vi "Replace-action.vi"(8 "error in (no error)":errorcluster, 9 "Position in":i32, 10 "Action":refnum<class "Action.lvclass">, 11 "Sequence in":refnum<class "Action-sequence.lvclass">) -> (0 "error out":errorcluster, 1 "Position":i32, 2 "Replaced action":refnum<class "Action.lvclass">, 3 "Sequence out":refnum<class "Action-sequence.lvclass">)   [LabVIEW 2013, in "PowderDeposition.lvlib" / "Action-sequence.lvclass"]
uses:
  Action-sequence.lvclass
  Action/Action.lvclass
  Action-sequence.lvclass/Action-sequence.ctl
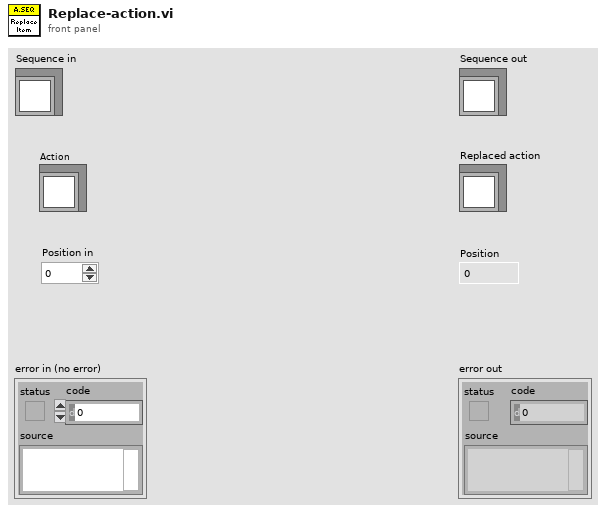
[diagram p1: front panel]
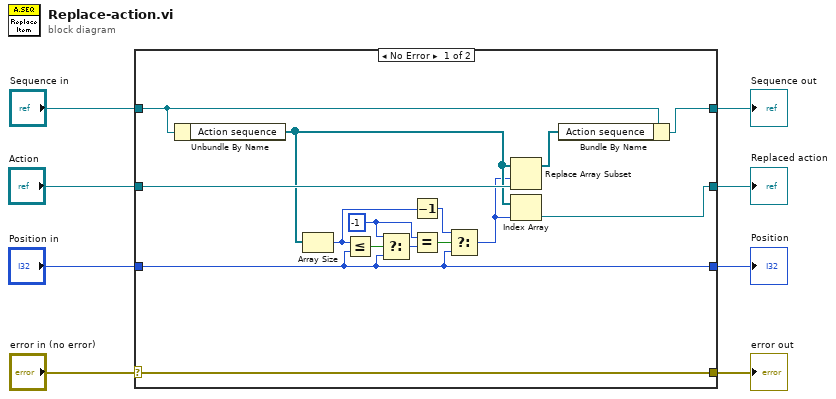
[diagram p0: block diagram]
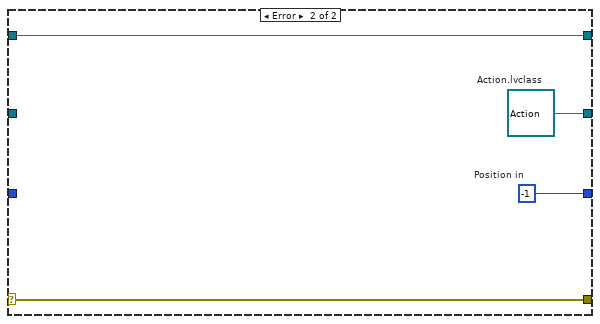
[diagram p2: hidden frame]
diagram:
  n1 = case shown="No Error" "error in (no error)" {
    selector: "error in (no error)" -> [w19 w27]
    tunnel: [w19 w27] -> w7
    tunnel: [w23 w26] -> w5
    tunnel: "Sequence in" -> [w22 w26]
    tunnel: "Action" -> [w20 _]
    tunnel: "Position in" -> [w10 _]
    tunnel: [w10 w25] -> w2
    tunnel: [w17 w24] -> w1
    frame No Error {
      w14 = -1 ("t")
      n2 = Unbundle By Name(w22) -> ("Action sequence"=w18:refnum<class "Action.lvclass">[])
      n3 = Array Size(array=w18) -> (size(s)=w11:i32)
      n4 = Less Or Equal?(x=w11, y=w10) -> (x <= y?=w16:bool)
      n5 = Select(t=w14, s=w16, f=w10) -> (s? t:f=w15:i32)
      n6 = Decrement(x=w11) -> (x-1=w12:i32)
      n7 = Equal?(x=w14, y=w15) -> (x = y?=w13:bool)
      n8 = Select(t=w12, s=w13, f=w10) -> (s? t:f=w9:i32)
      n9 = Replace Array Subset(array=w18, new element=w20, index=w9) -> (w21:refnum<class "Action.lvclass">[])
      n10 = Index Array(array=w18, index=w9) -> (element=w17:refnum<class "Action.lvclass">)
      n11 = Bundle By Name(cluster=w22, "Action sequence"=w21) -> (w23:refnum<class "Action-sequence.lvclass">)
    }
    frame Error {
      w24 = refnum<class "Action.lvclass"> refnum  # Action.lvclass
      w25 = -1  # Position in
    }
  }
  "error out" <- w7
  "Sequence out" <- w5
  "Position" <- w2
  "Replaced action" <- w1
